vi "CreateProduct.vi"(8 "Error In":errorcluster, 11 "reference in":refnum<class "SedanCarFactory.lvclass">) -> (0 "Error Out":errorcluster, 2 "ICarProduct":refnum<class "ICarProduct.lvclass">, 3 "reference out":refnum<class "SedanCarFactory.lvclass">)   [LabVIEW 2024, in "SedanCarFactory.lvclass"]
uses:
  SedanCarFactory.lvclass
  SedanCarFactory.lvclass/SedanCarFactory.ctl
  Sedan/Sedan.lvclass
  C:/Users/burakkorkmaz/Desktop/Leveling/labview-design-patterns/Factory Method Pattern/Labview/Sedan/Sedan.lvclass
  C:/Users/burakkorkmaz/Desktop/Leveling/labview-design-patterns/Factory Method Pattern/Labview/ICarProduct/ICarProduct.lvclass
  ICarProduct/ICarProduct.lvclass
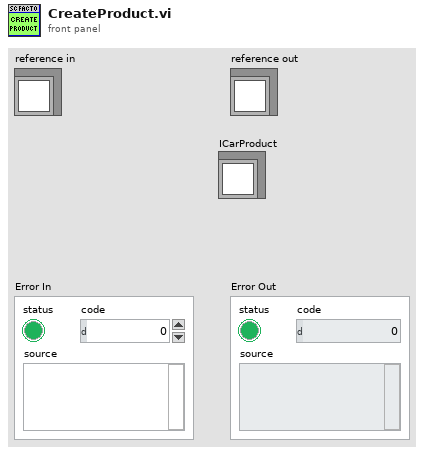
[diagram p1: front panel]
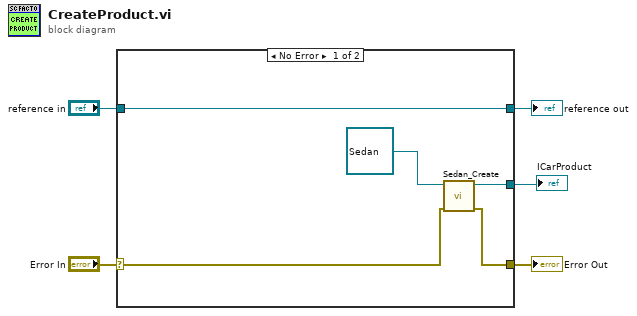
[diagram p0: block diagram]
diagram:
  n1 = case shown="No Error" "Error In" {
    selector: "Error In" -> [w8 w12]
    tunnel: [w7 w12] -> w4
    tunnel: [w10 w11] -> w2
    tunnel: "reference in" -> [w10 w11]
    tunnel: [w9 _] -> w1
    frame No Error {
      n2 = call "Sedan_Create.vi"("Error In"=w8, "reference in"=refnum<class "Sedan.lvclass"> refnum ("Sedan")) -> ("Error Out"=w7:errorcluster, "reference out"=w9:refnum<class "Sedan.lvclass">)  [unwired: 8 in]
    }
    frame Error {
    }
  }
  "Error Out" <- w4
  "reference out" <- w2
  "ICarProduct" <- w1
